vi "Weighted_Cross_Moments.vi"(0 "U":dbl[](array[numeric]) format="%.2f", 1 "W":dbl[](array[numeric]) format="%.2f", 2 "Block No":i32=1, 3 "Inst names":string[](array[string]), 5 "Shift in":dbl[](array[numeric]) format="%.2f", 6 "Weighting":dbl[](array[numeric]) format="%.2f", 8 "Indicies":i32[](array[numeric])) -> (14 "Correlations Only":string[](array[string]), 15 "All Results for file":string[](array[string]), 17 "Velocity Cluster Array Out":T1[](array[typedef]) {"u^4" format="%.2f"; "Mean % Err" format="%.2f"; "u^4/(u^2)^2 -3" format="%.2f"; "u^3/(u^2)^(1.5)" format="%.2f"; "u^2" format="%.2f"; "% u'/U" format="%.2f"; "U" format="%.2f"}, 19 "Shift out":dbl[](array[numeric]) format="%.2f")   [LabVIEW 2010]
uses:
  Controls/Velocity_cluster.ctl
  Globals/Meas_global.vi
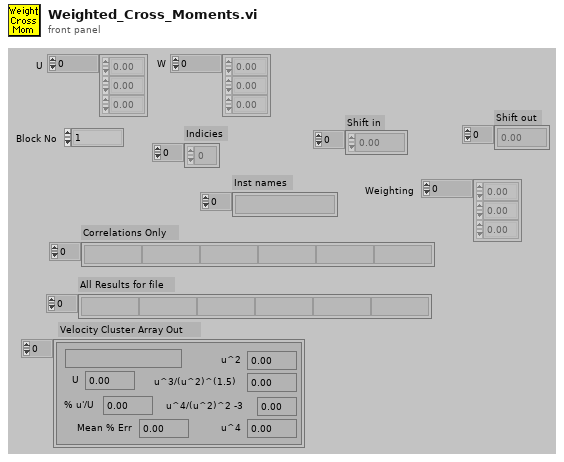
[diagram p1: front panel]
types:
  T1 = typedef "Velocity_cluster.ctl" = cluster{"Name":string, "U":dbl, "u^2":dbl, "u^3/(u^2)^(1.5)":dbl, "u^4/(u^2)^2 -3":dbl, "% u'/U":dbl, "Mean % Err":dbl, "u^4":dbl}
  T2 = typedef "Correlation_cluster.ctl" = cluster{"U inst":string, "W inst":string, "uw":dbl, "uw/u'w'":dbl, "u^2w":dbl, "uw^2":dbl, "uw^3":dbl, "u^3w":dbl, "u^2w^2":dbl}
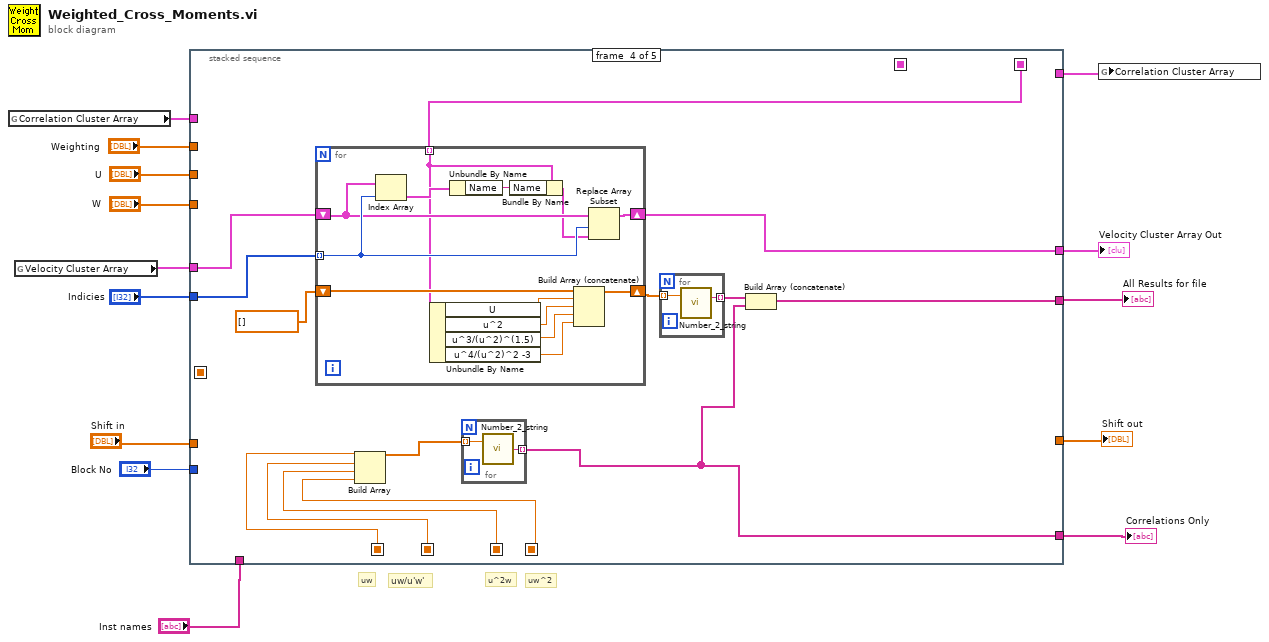
[diagram p0: block diagram]
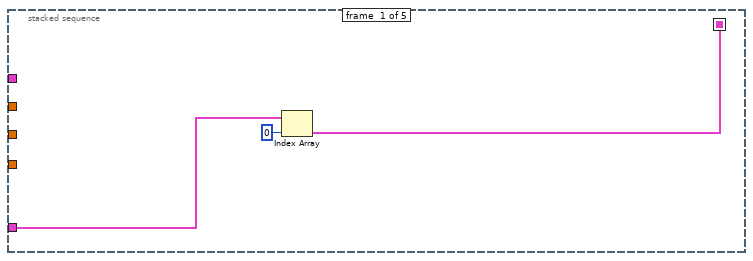
[diagram p2: hidden frame]
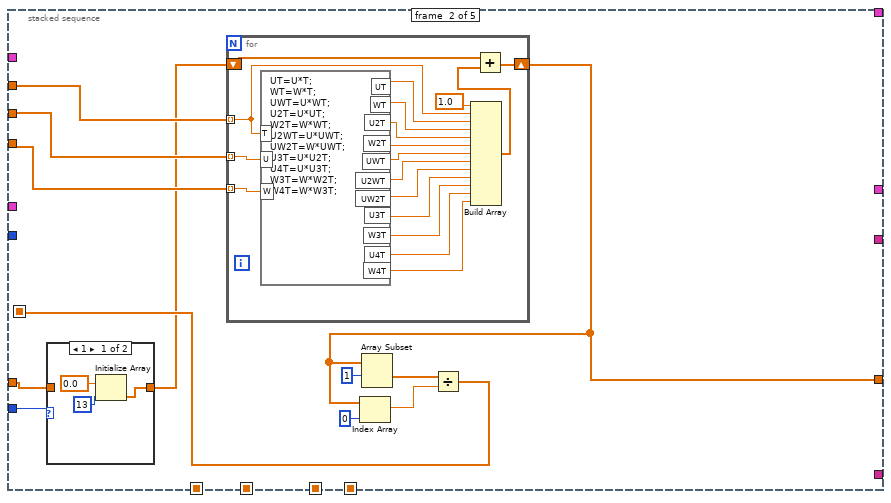
[diagram p3: hidden frame]
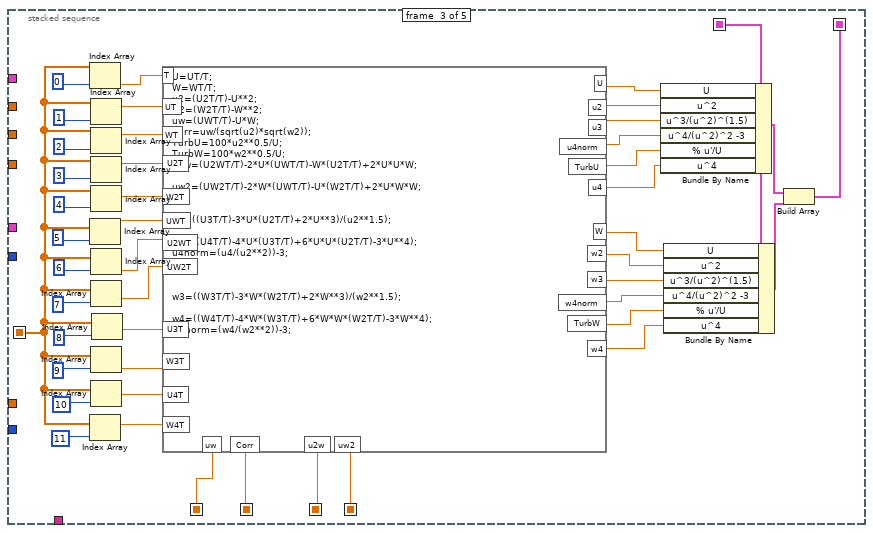
[diagram p5: hidden frame]
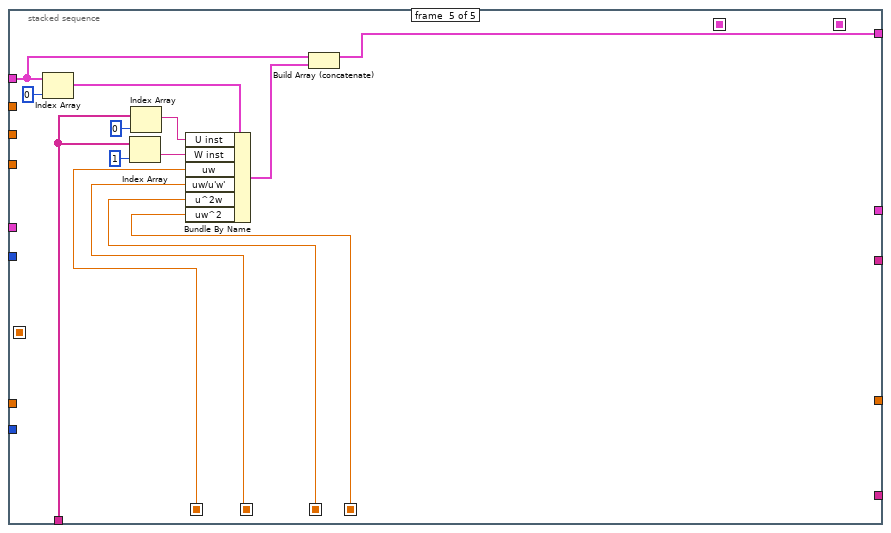
[diagram p6: hidden frame]
diagram:
  # "uw^2"
  # "u^2w"
  # "uw/u'w'"
  # "uw"
  n1 = global read "Meas_global.vi" "Correlation Cluster Array"() -> (w11:T2[])
  n2 = global read "Meas_global.vi" "Velocity Cluster Array"() -> (w2:T1[])
  n3 = stacked-sequence {
    seq-local: [_ _ w84 _ _] -> [_ _ _ w110 w140]
    seq-local: [_ _ w83 _ _] -> [_ _ _ w109 w139]
    seq-local: [_ w21 _ _ _] -> [_ _ w72 _ _]
    seq-local: [_ _ w78 _ _] -> [_ _ _ w108 w129]
    seq-local: [_ _ w77 _ _] -> [_ _ _ w107 w128]
    seq-local: [w15 _ _ _ _] -> [_ _ w67 _ _]
    seq-local: [_ _ w54 _ _] -> [_ _ _ w103 _]
    tunnel: "U" -> [_ w28 _ _ _]
    tunnel: [_ w22 _ _ _] -> w13
    tunnel: "Shift in" -> [_ w19 _ _ _]
    tunnel: [_ _ _ w97 _] -> w12
    tunnel: w11 -> [_ _ _ _ w137]
    tunnel: [_ _ _ _ w135] -> w10
    tunnel: "W" -> [_ w27 _ _ _]
    tunnel: "Inst names" -> [_ _ _ _ w132]
    tunnel: "Weighting" -> [_ w29 _ _ _]
    tunnel: w2 -> [w16 _ _ w106 _]
    tunnel: [_ _ _ w105 _] -> w1
    tunnel: "Indicies" -> [_ _ _ w104 _]
    tunnel: [_ _ _ w100 _] -> w5
    tunnel: "Block No" -> [_ w20 _ _ _]
    frame #0 {
      n4 = Index Array(array=w16, index=0 ("Index")) -> (element=w15:T1)
    }
    frame #1 {
      n5 = case shown="1" w20 {
        tunnel: [w30 w33] -> w18
        tunnel: w19 -> [_ w33]
        frame 1 {
          n6 = Initialize Array(0.0 ("Element Data"), 13 ("Dimension Size")) -> (w30:dbl[])
        }
        frame 2, Default {
        }
      }
      n7 = for {
        shift-right: [w39] -> w22
        shift-left: w18 -> [w51]
        tunnel: w29 -> [w49] mode=indexing
        tunnel: w28 -> [w48] mode=indexing
        tunnel: w27 -> [w47] mode=indexing
        n8 = formula code="UT=U*T;\nWT=W*T;\nUWT=U*WT;\nU2T=U*UT;\nW2T=W*WT;\nU2WT=U*UWT;\nUW2T=W*UWT;\nU3T=U*U2T;\nU4T=U*U3T;\nW3T=W*W2T;\nW4T=W*W3T;"("W"=w47, "U"=w48, "T"=w49) -> ("UWT"=w42:dbl, "UT"=w46:dbl, "WT"=w45:dbl, "U2T"=w44:dbl, "W2T"=w43:dbl, "U2WT"=w41:dbl, "UW2T"=w40:dbl, "U3T"=w38:dbl, "U4T"=w36:dbl, "W3T"=w37:dbl, "W4T"=w35:dbl)
        n9 = Build Array(1.0 ("Input Element"), w49, w46, w45, w44, w43, w42, w41, w40, w38, w37, w36, w35) -> (w50:dbl[])
        n10 = Add(x=w51, y=w50) -> (x+y=w39:dbl[])
      }
      n11 = Index Array(array=w22, index=0 ("Index")) -> (element=w23:dbl)
      n12 = Array Subset(array=w22, index=1 ("Array Index")) -> (w24:dbl[])  [unwired: 1 in]
      n13 = Divide(x=w24, y=w23) -> (x/y=w21:dbl[])
    }
    frame #2 {
      n14 = Index Array(array=w72, index=0) -> (element=w90:dbl)
      n15 = Index Array(array=w72, index=5) -> (element=w85:dbl)
      n16 = Index Array(array=w72, index=11) -> (element=w70:dbl)
      n17 = Index Array(array=w72, index=1) -> (element=w89:dbl)
      n18 = Index Array(array=w72, index=2) -> (element=w88:dbl)
      n19 = Index Array(array=w72, index=3) -> (element=w87:dbl)
      n20 = Index Array(array=w72, index=4) -> (element=w86:dbl)
      n21 = Index Array(array=w72, index=6) -> (element=w80:dbl)
      n22 = Index Array(array=w72, index=7) -> (element=w79:dbl)
      n23 = Index Array(array=w72, index=9) -> (element=w68:dbl)
      n24 = Index Array(array=w72, index=10) -> (element=w71:dbl)
      n25 = Index Array(array=w72, index=8) -> (element=w69:dbl)
      n26 = formula code="U=UT/T;\nW=WT/T;\nu2=(U2T/T)-U**2;\nw2=(W2T/T)-W**2;\nuw=(UWT/T)-U*W;\nCorr=uw/(sqrt(u2)*sqrt(w2));\nTurbU=100*u2**0.5/U;\nTurbW=100*w2**0.5/U;\nu2w=(U2WT/T)-2*U*(UWT/T)-W*(U2T/T)+2*U*U*W;\n\nuw2=(UW2T/T)-2*W*(UWT/T)-U*(W2T/T)+2*U*W*W;\n\n\nu3=((U3T/T)-3*U*(U2T/T)+2*U**3)/(u2**1.5);\n\nu4=((U4T/T)-4*U*(U3T/T)+6*U*U*(U2T/T)-3*U**4);\nu4norm=(u4/(u2**2))-3;\n\n\n\nw3=((W3T/T)-3*W*(W2T/T)+2*W**3)/(w2**1.5);\n\nw4=((W4T/T)-4*W*(W3T/T)+6*W*W*(W2T/T)-3*W**4);\nw4norm=(w4/(w2**2))-3;"("T"=w90, "UT"=w89, "WT"=w88, "W2T"=w86, "UWT"=w85, "U2T"=w87, "U2WT"=w80, "UW2T"=w79, "U3T"=w69, "U4T"=w71, "W3T"=w68, "W4T"=w70) -> ("uw"=w84:dbl, "U"=w60:dbl, "W"=w65:dbl, "u2"=w57:dbl, "w2"=w64:dbl, "Corr"=w83:dbl, "u2w"=w78:dbl, "uw2"=w77:dbl, "u3"=w58:dbl, "u4norm"=w59:dbl, "w3"=w63:dbl, "w4norm"=w62:dbl, "TurbU"=w66:dbl, "TurbW"=w61:dbl, "w4"=w52:dbl, "u4"=w53:dbl)
      n27 = Bundle By Name(cluster=w67, "U"=w60, "u^2"=w57, "u^3/(u^2)^(1.5)"=w58, "u^4/(u^2)^2 -3"=w59, "% u'/U"=w66, "u^4"=w53) -> (w55:T1)
      n28 = Bundle By Name(cluster=w67, "U"=w65, "u^2"=w64, "u^3/(u^2)^(1.5)"=w63, "u^4/(u^2)^2 -3"=w62, "% u'/U"=w61, "u^4"=w52) -> (w56:T1)
      n29 = Build Array(w55, w56) -> (w54:T1[])
    }
    frame #3 {
      n30 = for {
        shift-right: [w127] -> w105
        shift-left: w106 -> [w117]
        tunnel: w104 -> [w118] mode=indexing
        tunnel: w103 -> [w115] mode=indexing
        shift-right: [w125] -> w99
        shift-left: dbl[] [] -> [w126]
        n31 = Index Array(array=w117, index=w118) -> (element=w120:T1)
        n32 = Unbundle By Name(w115) -> ("U"=w124:dbl, "u^2"=w123:dbl, "u^3/(u^2)^(1.5)"=w122:dbl, "u^4/(u^2)^2 -3"=w121:dbl)
        n33 = Unbundle By Name(w120) -> ("Name"=w119:string)
        n34 = Bundle By Name(cluster=w115, "Name"=w119) -> (w116:T1)
        n35 = Build Array (concatenate)(w126, w124, w123, w122, w121) -> (w125:dbl[])
        n36 = Replace Array Subset(array=w117, new element=w116, index=w118) -> (w127:T1[])
      }
      n37 = Build Array(w110, w109, w108, w107) -> (w98:dbl[])
      n38 = for {
        tunnel: w98 -> [w112] mode=indexing
        tunnel: [w111] -> w97 mode=indexing
        n39 = call "Number_2_string.vi"("number"=w112) -> ("String"=w111:string)  [unwired: 1 in]
      }
      n40 = for {
        tunnel: w99 -> [w114] mode=indexing
        tunnel: [w113] -> w101 mode=indexing
        n41 = call "Number_2_string.vi"("number"=w114) -> ("String"=w113:string)  [unwired: 1 in]
      }
      n42 = Build Array (concatenate)(w101, w97) -> (w100:string[])
    }
    frame #4 {
      n43 = Index Array(array=w137, index=0) -> (element=w141:T2)
      n44 = Index Array(array=w132, index=1) -> (element=w130:string)
      n45 = Index Array(array=w132, index=0) -> (element=w131:string)
      n46 = Bundle By Name(cluster=w141, "U inst"=w131, "W inst"=w130, "uw"=w140, "uw/u'w'"=w139, "u^2w"=w129, "uw^2"=w128) -> (w136:T2)
      n47 = Build Array (concatenate)(w137, w136) -> (w135:T2[])
    }
  }
  "Shift out" <- w13
  "Correlations Only" <- w12
  "All Results for file" <- w5
  "Velocity Cluster Array Out" <- w1
  n48 = global write "Meas_global.vi" "Correlation Cluster Array"(w10) -> ()
